vi "QueryHardware.vi"(8 "error in (no error)":errorcluster, 11 "Target Reference In":refnum<k39>) -> (0 "error out":errorcluster, 2 "Chassis List out":T1[](array[typedef]), 3 "Target Reference out":refnum<k39>)   [LabVIEW 2027, in "VeriStandTestUtilities.lvlib"]
uses:
  VeriStandTestUtilities.lvlib
  C:/NetCoreDLL/NationalInstruments.VeriStand.SystemDefinitionAPI.dll
  NetCoreDLL/NationalInstruments.VeriStand.SystemDefinitionAPI.dll
  ChassisInformation.ctl
panel:
  in  "Cluster":T1
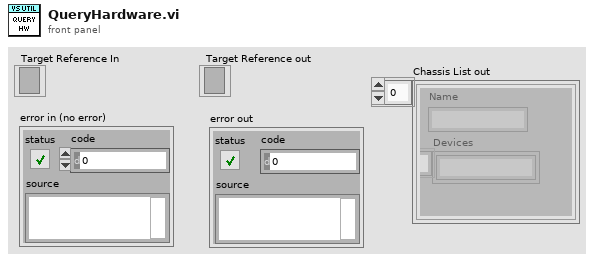
[diagram p1: front panel]
types:
  T1 = typedef "VeriStandTestUtilities.lvlib/ChassisInformation.ctl" = cluster{"Name":string, "Devices":string[]}
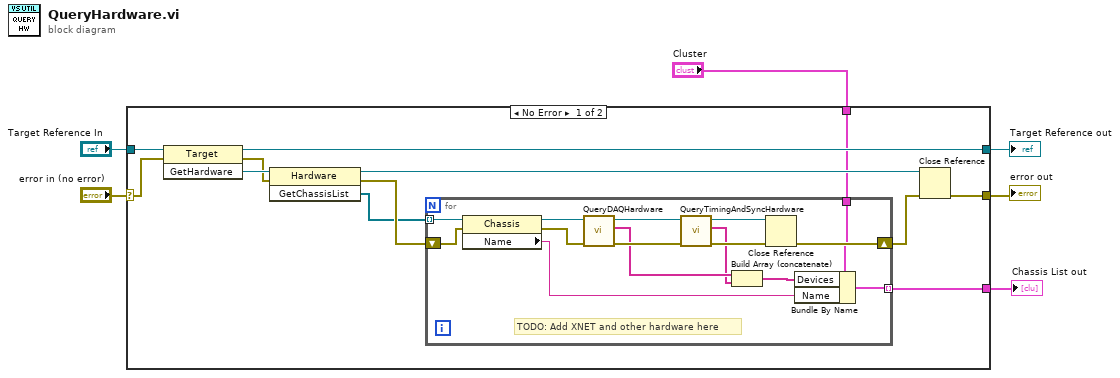
[diagram p0: block diagram]
diagram:
  n1 = case shown="No Error" "error in (no error)" {
    selector: "error in (no error)" -> [w13 w35]
    tunnel: [w10 w35] -> w5
    tunnel: "Target Reference In" -> [w15 w34]
    tunnel: [w11 w34] -> w3
    tunnel: "Cluster" -> [w8 _]
    tunnel: [w7 _] -> w1
    frame No Error {
      n2 = invoke class="Target" method="GetHardware"(reference=w15, error in=w13) -> (reference out=w11:refnum<k39>, error out=w17:errorcluster, "GetHardware"=w18:refnum<k39>)  [unwired: 1 in]
      n3 = invoke class="Hardware" method="GetChassisList"(reference=w18, error in=w17) -> (reference out=w14:refnum<k39>, error out=w16:errorcluster, "GetChassisList"=w9:refnum<k39>[])  [unwired: 1 in]
      n4 = for {
        shift-right: [w33] -> w12
        shift-left: w16 -> [w24]
        tunnel: w9 -> [w26] mode=indexing
        tunnel: w8 -> [w22]
        tunnel: [w19] -> w7 mode=indexing
        # "TODO: Add XNET and other hardware here"
        n5 = property class="Chassis"(reference=w26, error in=w24) -> (reference out=w25:refnum<k39>, error out=w23:errorcluster, "Name"=w21:string)
        n6 = call "QueryDAQHardware.vi"("error in (no error)"=w23, "NationalInstruments.VeriStand.SystemDefinitionAPI.Chassis"=w25) -> ("error out"=w30:errorcluster, "Devices out"=w28:string[], "NationalInstruments.VeriStand.SystemDefinitionAPI.Chassis"=w32:refnum<k39>)  [unwired: 7 in]
        n7 = call "QueryTimingAndSyncHardware.vi"("error in (no error)"=w30, "NationalInstruments.VeriStand.SystemDefinitionAPI.Chassis"=w32) -> ("error out"=w29:errorcluster, "Devices out"=w27:string[], "NationalInstruments.VeriStand.SystemDefinitionAPI.Chassis"=w31:refnum<k39>)  [unwired: 7 in]
        n8 = Build Array (concatenate)(w28, w27) -> (w20:string[])
        n9 = Close Reference(reference=w31, error in (no error)=w29) -> (error out=w33:errorcluster)
        n10 = Bundle By Name(cluster=w22, "Devices"=w20, "Name"=w21) -> (w19:T1)
      }
      n11 = Close Reference(reference=w14, error in (no error)=w12) -> (error out=w10:errorcluster)
    }
    frame Error {
    }
  }
  "Target Reference out" <- w3
  "error out" <- w5
  "Chassis List out" <- w1
